vi "Refnum Names.vi"() -> ()   [LabVIEW 2017]
panel:
  in  "Intake Out":string="Intake Out"
  in  "Compressor":string="Compressor"
  in  "RPED Right":string="RPED Right"
  in  "Intake Rotation Lower Limit Switch":string="Intake Rotation Lower Limit Swtich"
  in  "Cube IR":string="Lift Upper Limit Cube IR"
  in  "Lift Lower Limit Switch":string="Lift Lower Limit Switch"
  in  "Lift Upper Limit Switch":string="Lift Upper Limit Switch"
  in  "Intake Rotation Upper Limit Switch":string="Intake Rotation Upper Limit Swtich"
  in  "Pigeon IMU":string="Pigeon IMU"
  in  "RPED Left":string="RPED Left"
  in  "Intake Motor":string="Intake Motor"
  in  "Brake":string="Brake"
  in  "Intake":string="Intake"
  in  "Drive Shift":string="Drive Shift"
  in  "Arm Rotation":string="Arm Rotation"
  in  "LED CANifier":string="LED CANifier"
  in  "LED Set Notifier":string="LED Set Notifier"
  in  "LED Execute Notifier":string="LED Execute Notifier"
  in  "Lift Slave":string="Lift Slave"
  in  "Lift Master":string="Lift Master"
  in  "Right Drive Slave 2":string="Right Drive Slave 2"
  in  "Right Drive Slave 1":string="Right Drive Slave 1"
  in  "Right Drive Master":string="Right Drive Master"
  in  "Left Drive Slave 2":string="Left Drive Slave 2"
  in  "Left Drive Slave 1":string="Left Drive Slave 1"
  in  "Left Drive Master":string="Left Drive Master"
  in  "Intake Rotation Set Notifier":string="Intake_Rotation Set Notifier"
  in  "Intake Rotation Execute Notifier":string="Intake_Rotation  Execute Notifier"
  in  "RPED Set Notifier":string="RPED Set Notifier"
  in  "RPED Execute Notifier":string="RPED Execute Notifier"
  in  "Lift Set Notifier":string="Lift Set Notifier"
  in  "Lift Execute Notifier":string="Lift Execute Notifier"
  in  "Intake Set Notifier":string="Intake Set Notifier"
  in  "Intake Execute Notifier":string="Intake Execute Notifier"
  in  "Drive Set Notifier":string="Drive Set Notifier"
  in  "Drive Execute Notifier":string="Drive Execute Notifier"
  in  "CoPilot Controller":string="CoPilot Controller"
  in  "Pilot Controller":string="Pilot Controller"
  # "Notifiers"
  # "Motors"
  # "Sensors"
  # "Pneumatics"
  # "Third state (forced open)\nof arm pneumatic"
  # "Closed state of arm pneumatic"
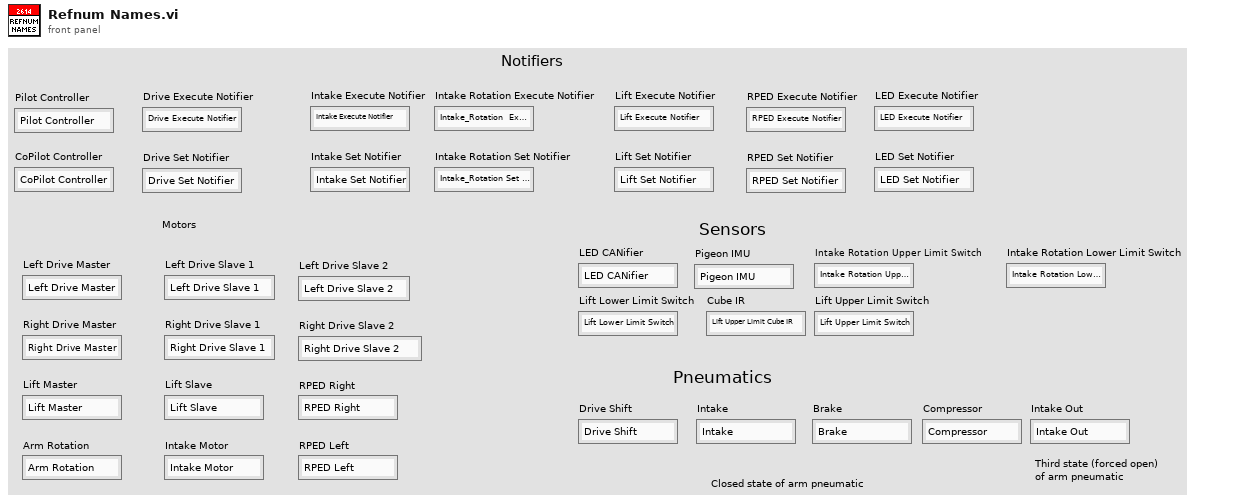
[diagram p1: front panel]
diagram:
